vi "Scale_0-25mm_to-0-5vdc.vi"(8 "error in (no error)":errorcluster, 11 "Input (mm)":dbl=1.0 caption="m") -> (0 "error out":errorcluster, 3 "Output (vdc)":dbl)   [LabVIEW 2018]
doc: "Changes the amplitude of a signal by scaling or mapping the signal.\n--------------------\n\nThis Express VI is configured as follows:\n\nScaling Type: Interpolated"
uses:
  <vilib>/express/express shared/scalingTypes.ctl
panel:
  in  "Lowest Peak":dbl
  in  "Highest Peak":dbl=1.0
  in  "dB Reference":dbl=1.0
  in  "m":dbl=1.0
  in  "b":dbl
  in  "Scaling Type":T1=enum."Interpolation"
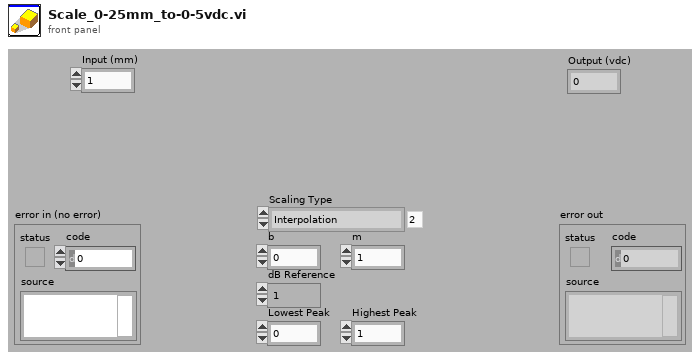
[diagram p1: front panel]
types:
  T1 = typedef "scalingTypes.ctl" = enum16{"Normalize", "Linear", "Interpolation", "Logarithmic"}
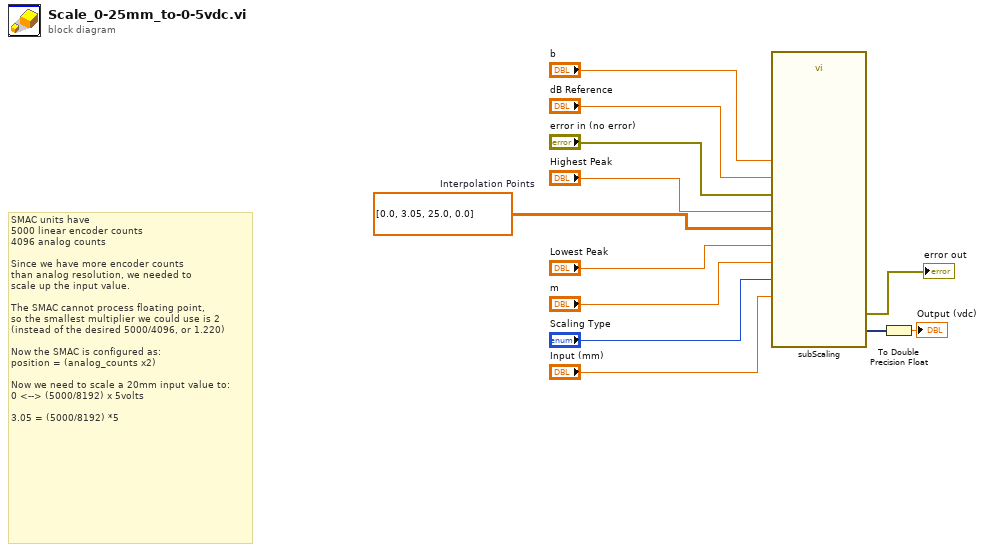
[diagram p0: block diagram]
diagram:
  w9 = dbl[][] [[0.0, 3.05], [25.0, 0.0]]  # Interpolation Points
  # "SMAC units have\n5000 linear encoder counts\n4096 analog counts\n\nSince we have more encoder counts\nthan analog resolution, we needed to\nscale up the input value.\n\nThe SMAC cannot process floating point,\nso the smallest multiplier we could use is 2 \n(instead of the desired 5000/4096, or 1.220)\n\nNow the SMAC is configured as:\nposition = (analog_counts x2)\n\nNow we need to scale a 20mm input value to:\n0 <--> (5000/8192) x 5volts\n\n3.05 = (5000/8192) *5"
  n1 = call <vilib>:"subScaling.vi"("Signals"="Input (mm)", "b"="b", "m"="m", "dB reference"="dB Reference", "Scaling Type"="Scaling Type", "error in (no error)"="error in (no error)", "Interpolation Points"=w9, "Highest Peak"="Highest Peak", "Lowest Peak"="Lowest Peak") -> ("Scaled Signals"=w3:dynamicdata, "error out"=→"error out":errorcluster)  [unwired: 5 in]
  n2 = To Double Precision Float(number=w3) -> (double precision float=→"Output (vdc)":dbl)
